vi "TestDiscovery.vi"(8 "error in (no error)":errorcluster, 11 "TestRunner in":refnum<class "TestRunner.lvclass">) -> (0 "error out":errorcluster, 3 "TestRunner out":refnum<class "TestRunner.lvclass">)   [LabVIEW 2019, in "TestRunner.lvlib" / "TestRunner.lvclass"]
uses:
  TestRunner.lvclass
  C:/Program Files (x86)/National Instruments/LabVIEW 2019/vi.lib/NI/Event Source Actor/Event Source/Event Source/Event Source.lvclass
  TestRunnerEvent.lvclass
  C:/Program Files (x86)/National Instruments/LabVIEW 2019/vi.lib/NI/Event Source Actor/Event Source/Event/Event.lvclass
  <vilib>/NI/Event Source Actor/Event Source/Event/Event.lvclass/Event.ctl
  <vilib>/NI/Event Source Actor/Event Source/Event/Event.lvclass
  <vilib>/NI/Event Source Actor/Event Source/Event Source/Event Source.lvclass
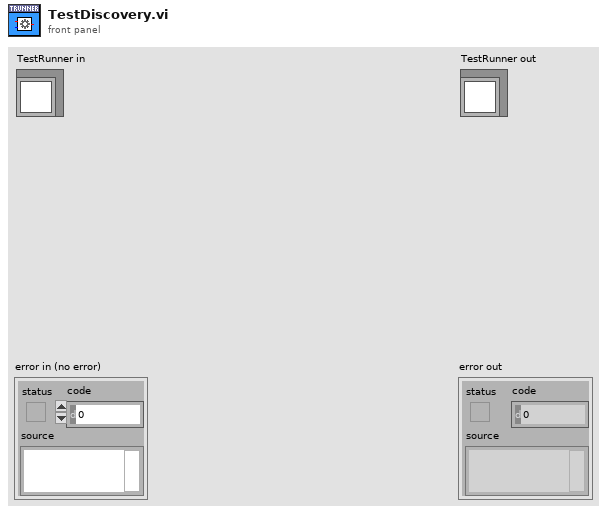
[diagram p1: front panel]
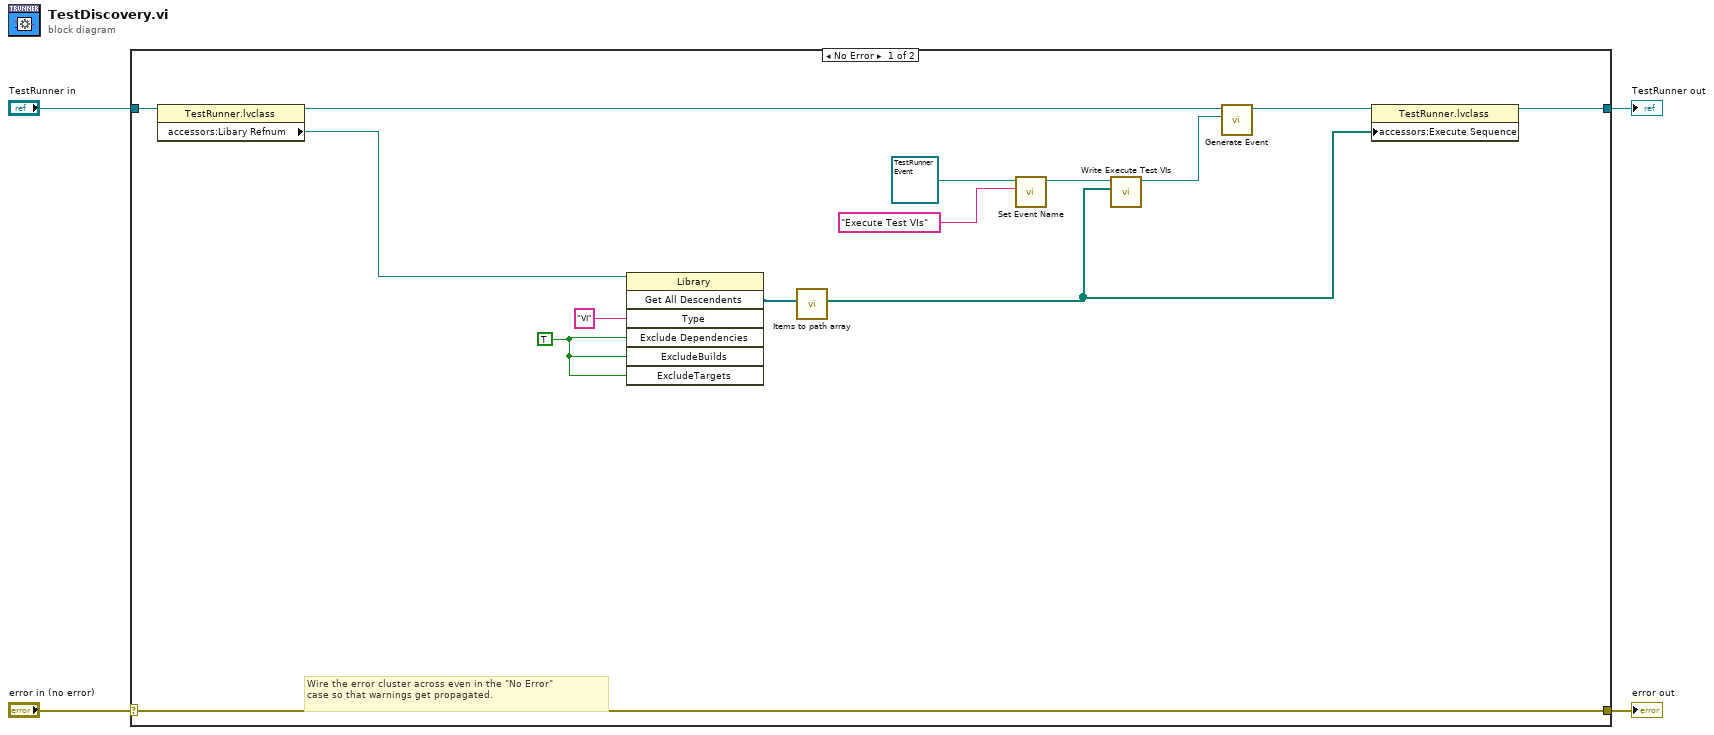
[diagram p0: block diagram]
diagram:
  n1 = case shown="No Error" "error in (no error)" {
    selector: "error in (no error)" -> [w18 w20]
    tunnel: [w18 w20] -> w3
    tunnel: [w17 w19] -> w1
    tunnel: "TestRunner in" -> [w10 w19]
    frame No Error {
      w6 = TRUE ("ExcludeDependencies")
      # "Wire the error cluster across even in the \"No Error\"\ncase so that warnings get propagated."
      n2 = property class="TestRunner.lvclass"(reference=w10) -> (reference out=w9:refnum<class "TestRunner.lvclass">, "accessors:Libary Refnum"=w5:refnum<vi>)  [unwired: 1 in, 1 out]
      n3 = invoke class="Library" method="Get All Descendents"(reference=w5, "Type"="VI", "Exclude Dependencies"=w6, "ExcludeBuilds"=w6, "ExcludeTargets"=w6) -> ("All Descendents"=w7:refnum<vi>[])  [unwired: 2 in, 6 out]
      n4 = call "Items to path array.vi"("Project Items"=w7) -> ("Paths"=w13:path[])  [unwired: 10 in]
      n5 = call <vilib>:"Set Event Name.vi"("Name (Generic)"="Execute Test VIs", "Event In"=refnum<class "TestRunnerEvent.lvclass"> refnum ("UnitTestEngine.lvlib:TestRunnerEvent.lvclass")) -> ("Event Out"=w14:refnum<class "TestRunnerEvent.lvclass">)  [unwired: 9 in]
      n6 = call-dynamic "Write Execute Test VIs.vi"("Execute Test VIs"=w13, "TestRunnerEvent in"=w14) -> ("TestRunnerEvent out"=w11:refnum<class "TestRunnerEvent.lvclass">)  [unwired: 8 in, 1 out]
      n7 = call <vilib>:"Generate Event.vi"("Event"=w11, "Event Source In"=w9) -> ("Event Source Out"=w12:refnum<class "TestRunner.lvclass">)  [unwired: 8 in, 1 out]
      n8 = property class="TestRunner.lvclass"(reference=w12, "accessors:Execute Sequence"=w13) -> (reference out=w17:refnum<class "TestRunner.lvclass">)  [unwired: 1 in, 1 out]
    }
    frame Error {
    }
  }
  "error out" <- w3
  "TestRunner out" <- w1
